vi "ex_3.vi"() -> ()   [LabVIEW 2020]
panel:
  out "Numeric 2":i32
  out "Numeric":i32
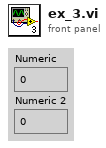
[diagram p1: front panel]
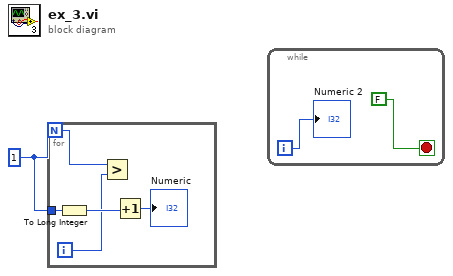
[diagram p0: block diagram]
diagram:
  w1 = 1
  n1 = for {
    N: w1 -> [w3]
    tunnel: w1 -> [w6]
    i -> [w2]
    n2 = To Long Integer(number=w6) -> (32bit integer=w4:i32)
    n3 = Greater?(x=w3, y=w2) -> ()  [unwired: 1 out]
    n4 = Increment(x=w4) -> (x+1=→"Numeric":i32)
  }
  n5 = while {
    i -> [w8]
    stop <- FALSE ("stop") stop-if-true
    "Numeric 2" <- w8
  }
